vi "test-DiffDrvPoseEst2-Test2.vi"(8 "error in (no error)":errorcluster) -> (0 "error out":errorcluster, 3 "Test Passed":bool)   [LabVIEW 2019]
uses:
  <vilib>/Rock Robotics/WPI/ThirdParty/JAS_Junk/TrajLib/Rotation2d_CreateAngle.vi
  <vilib>/Rock Robotics/WPI/ThirdParty/JAS_Junk/TrajLib/MatBuilder_Create.vi
  <vilib>/Rock Robotics/SystemInterfaces/NetworkCommunication/NetComm_UsageReport_report.vi
  <vilib>/Rock Robotics/WPI/ThirdParty/JAS_Junk/TrajLib/Pose2d_TransformBy.vi
  <vilib>/Rock Robotics/WPI/ThirdParty/JAS_Junk/TrajLib/Translation2d_RotateBy.vi
  <vilib>/Rock Robotics/WPI/ThirdParty/JAS_Junk/TrajLib/Translation2d_Plus.vi
  <vilib>/Rock Robotics/WPI/ThirdParty/JAS_Junk/TrajLib/Rotation2d_Plus.vi
  <vilib>/Rock Robotics/WPI/ThirdParty/JAS_Junk/TrajLib/Pose2d_New_TRRO.vi
  <vilib>/Rock Robotics/WPI/ThirdParty/JAS_Junk/TrajLib/Rotation2d_RotateBy.vi
  <vilib>/Rock Robotics/WPI/ThirdParty/JAS_Junk/TrajLib/Rotation2d_CreateXY.vi
  <vilib>/Rock Robotics/WPI/ThirdParty/JAS_Junk/TrajLib/Util_CalcDist.vi
  <vilib>/Rock Robotics/WPI/ThirdParty/JAS_Junk/TrajLib/Globals/Util_LibraryGlobals.vi
  <vilib>/Rock Robotics/WPI/ThirdParty/JAS_Junk/TrajLib/Trajectory_Library.lvlib
panel:
  out "max x error":dbl
  out "max y err":dbl
  out "Y Error":dbl[](array[numeric])
  out "X error":dbl[](array[numeric])
  out "Total":i32
  out "Total passed":i32
  out "Sub error":bool
  out "End Y pos passed":bool
  out "End X pos passed":bool
  out "AddVisionCount":i32
  out "TotalTImeSecs 2":dbl
  out "BenchProcessing \nTimer Per Pass":dbl
  out "BenchTotalTime":dbl
  out "BenchTotalPasses":dbl
  out "MaxErrPassed":bool
  out "MeanPassed":bool
  out "ErrorSumNormalized":dbl
  out "Error Sum":dbl
  out "Max Error":dbl
  out "VIsionMeasCount":i32
  out "TotalTImeSecs":dbl
  out "Position Graph":cluster{dbl[], dbl[]}[](graph)
  out "PoseEst2NewErr":errorcluster
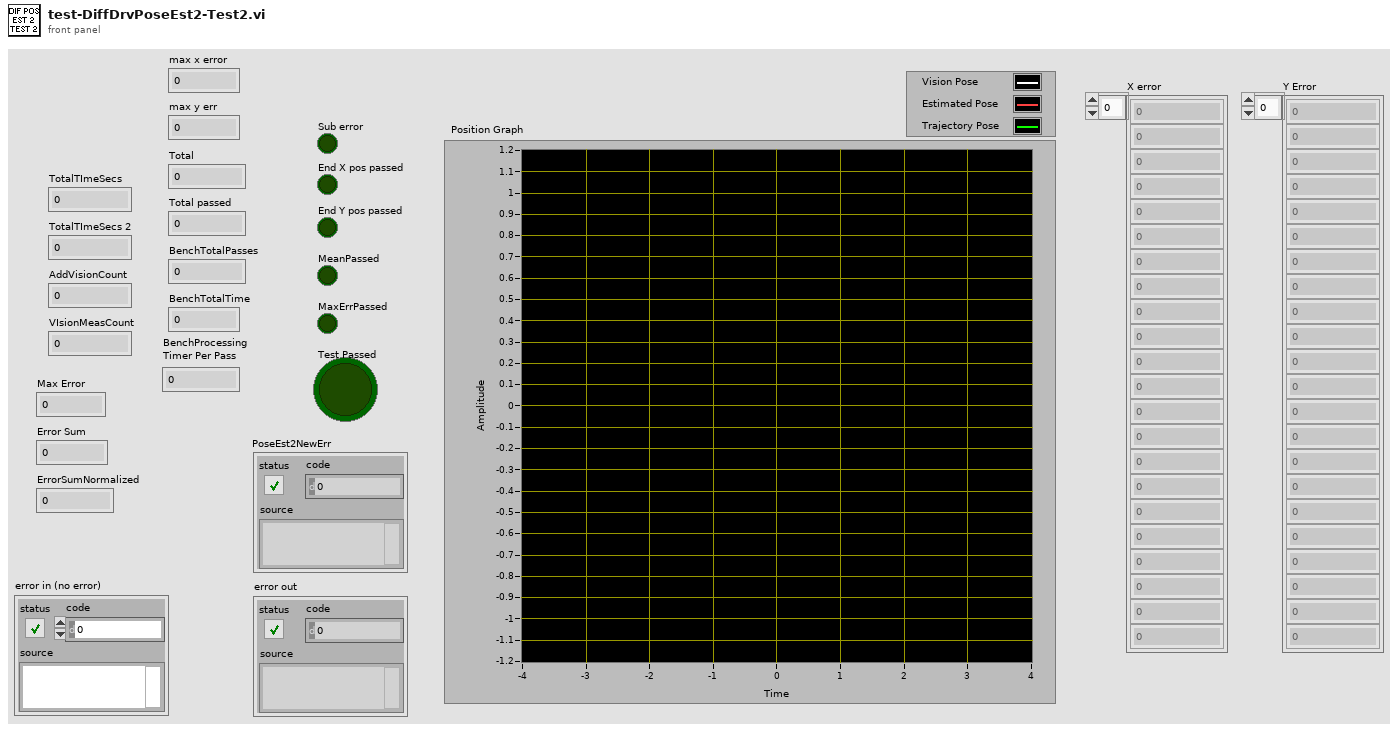
[diagram p1: front panel]
types:
  T1 = typedef "Trajectory_Library.lvlib/POSE2D.ctl" = cluster{"TRANSLATION":T2, "ROTATION":T3}
  T2 = typedef "Trajectory_Library.lvlib/TRANSLATION2D.ctl" = cluster{"X":dbl, "Y":dbl}
  T3 = typedef "Trajectory_Library.lvlib/ROTATION2D.ctl" = cluster{"VALUE":dbl, "COS":dbl, "SIN":dbl}
  T4 = typedef "NI_Matrix.lvlib/RealMatrix.ctl" = dbl[][]
  T5 = typedef "Trajectory_Library.lvlib/TRAJ_CONFIG.ctl" = cluster{"MaxVelocity":dbl, "Max Acceleration":dbl, "StartVelocity":dbl, "End Velocity":dbl, "Reversed":bool, "Constraints":variant[]}
  T6 = typedef "Trajectory_Library.lvlib/DIFF_DRIVE_KINEMATICS.ctl" = cluster{"TrackWidth_Meters":dbl}
  T7 = typedef "Trajectory_Library.lvlib/DIFF_DRIVE_POSE_EST2.ctl" = cluster{"M_Vision_K":T4, "m_nominal_dT":dbl, "m_PrevTime_Sec":dbl, "Pose_Buffer":T8, "Diff_Drive_Kinematics":T6, "Diff_Drive_Odom_2":T9, "M_Q":T4}
  T8 = typedef "Trajectory_Library.lvlib/TIME_INTERPOLATABLE_VARIANT.ctl" = cluster{"TimeStamps":dbl[], "DataArray":variant[], "Min_TimeStamp":dbl, "Max_TimeStamp":dbl, "ItemCount":i32, "MaxBufferTime":dbl}
  T9 = typedef "Trajectory_Library.lvlib/DIFF_DRIVE_ODOM2.ctl" = cluster{"M_POSE_Meters":T1, "M_GyroOffset":T3, "M_PrevAngle":T3, "M_PrevLeftDist_M":dbl, "M_PrevRightDist_M":dbl, "M_InitLeftDist_M":dbl, "M_InitRightDist_M":dbl}
  T10 = typedef "Trajectory_Library.lvlib/TRAJECTORY.ctl" = cluster{"TotalTImeSecs":dbl, "States":T11[]}
  T11 = typedef "Trajectory_Library.lvlib/TRAJ_STATE.ctl" = cluster{"TimeSeconds":dbl, "Velocity":dbl, "Acceleration":dbl, "POSE":T1, "Curvature":dbl}
  T12 = typedef "Trajectory_Library.lvlib/TRANSFORM2D.ctl" = cluster{"TRANSLATION":T2, "ROTATION":T3, "xF":bool}
  T13 = cluster{"MaxErrPassed":bool, "MeanPassed":bool, "Error Sum":dbl, "ErrorSumNormalized":dbl, "Max Error":dbl, "AddVisionCount":i32, "VIsionApplyCount":i32, "BenchTotalPasses":dbl, "BenchTotalTime":dbl, "BenchProcessing \nTimer Per Pass":dbl, "TotalTImeSecs":dbl, "End X pos passed":bool, "End Y pos passed":bool, "Sub error":bool, "End X Dev":dbl, "End Y Dev":dbl}
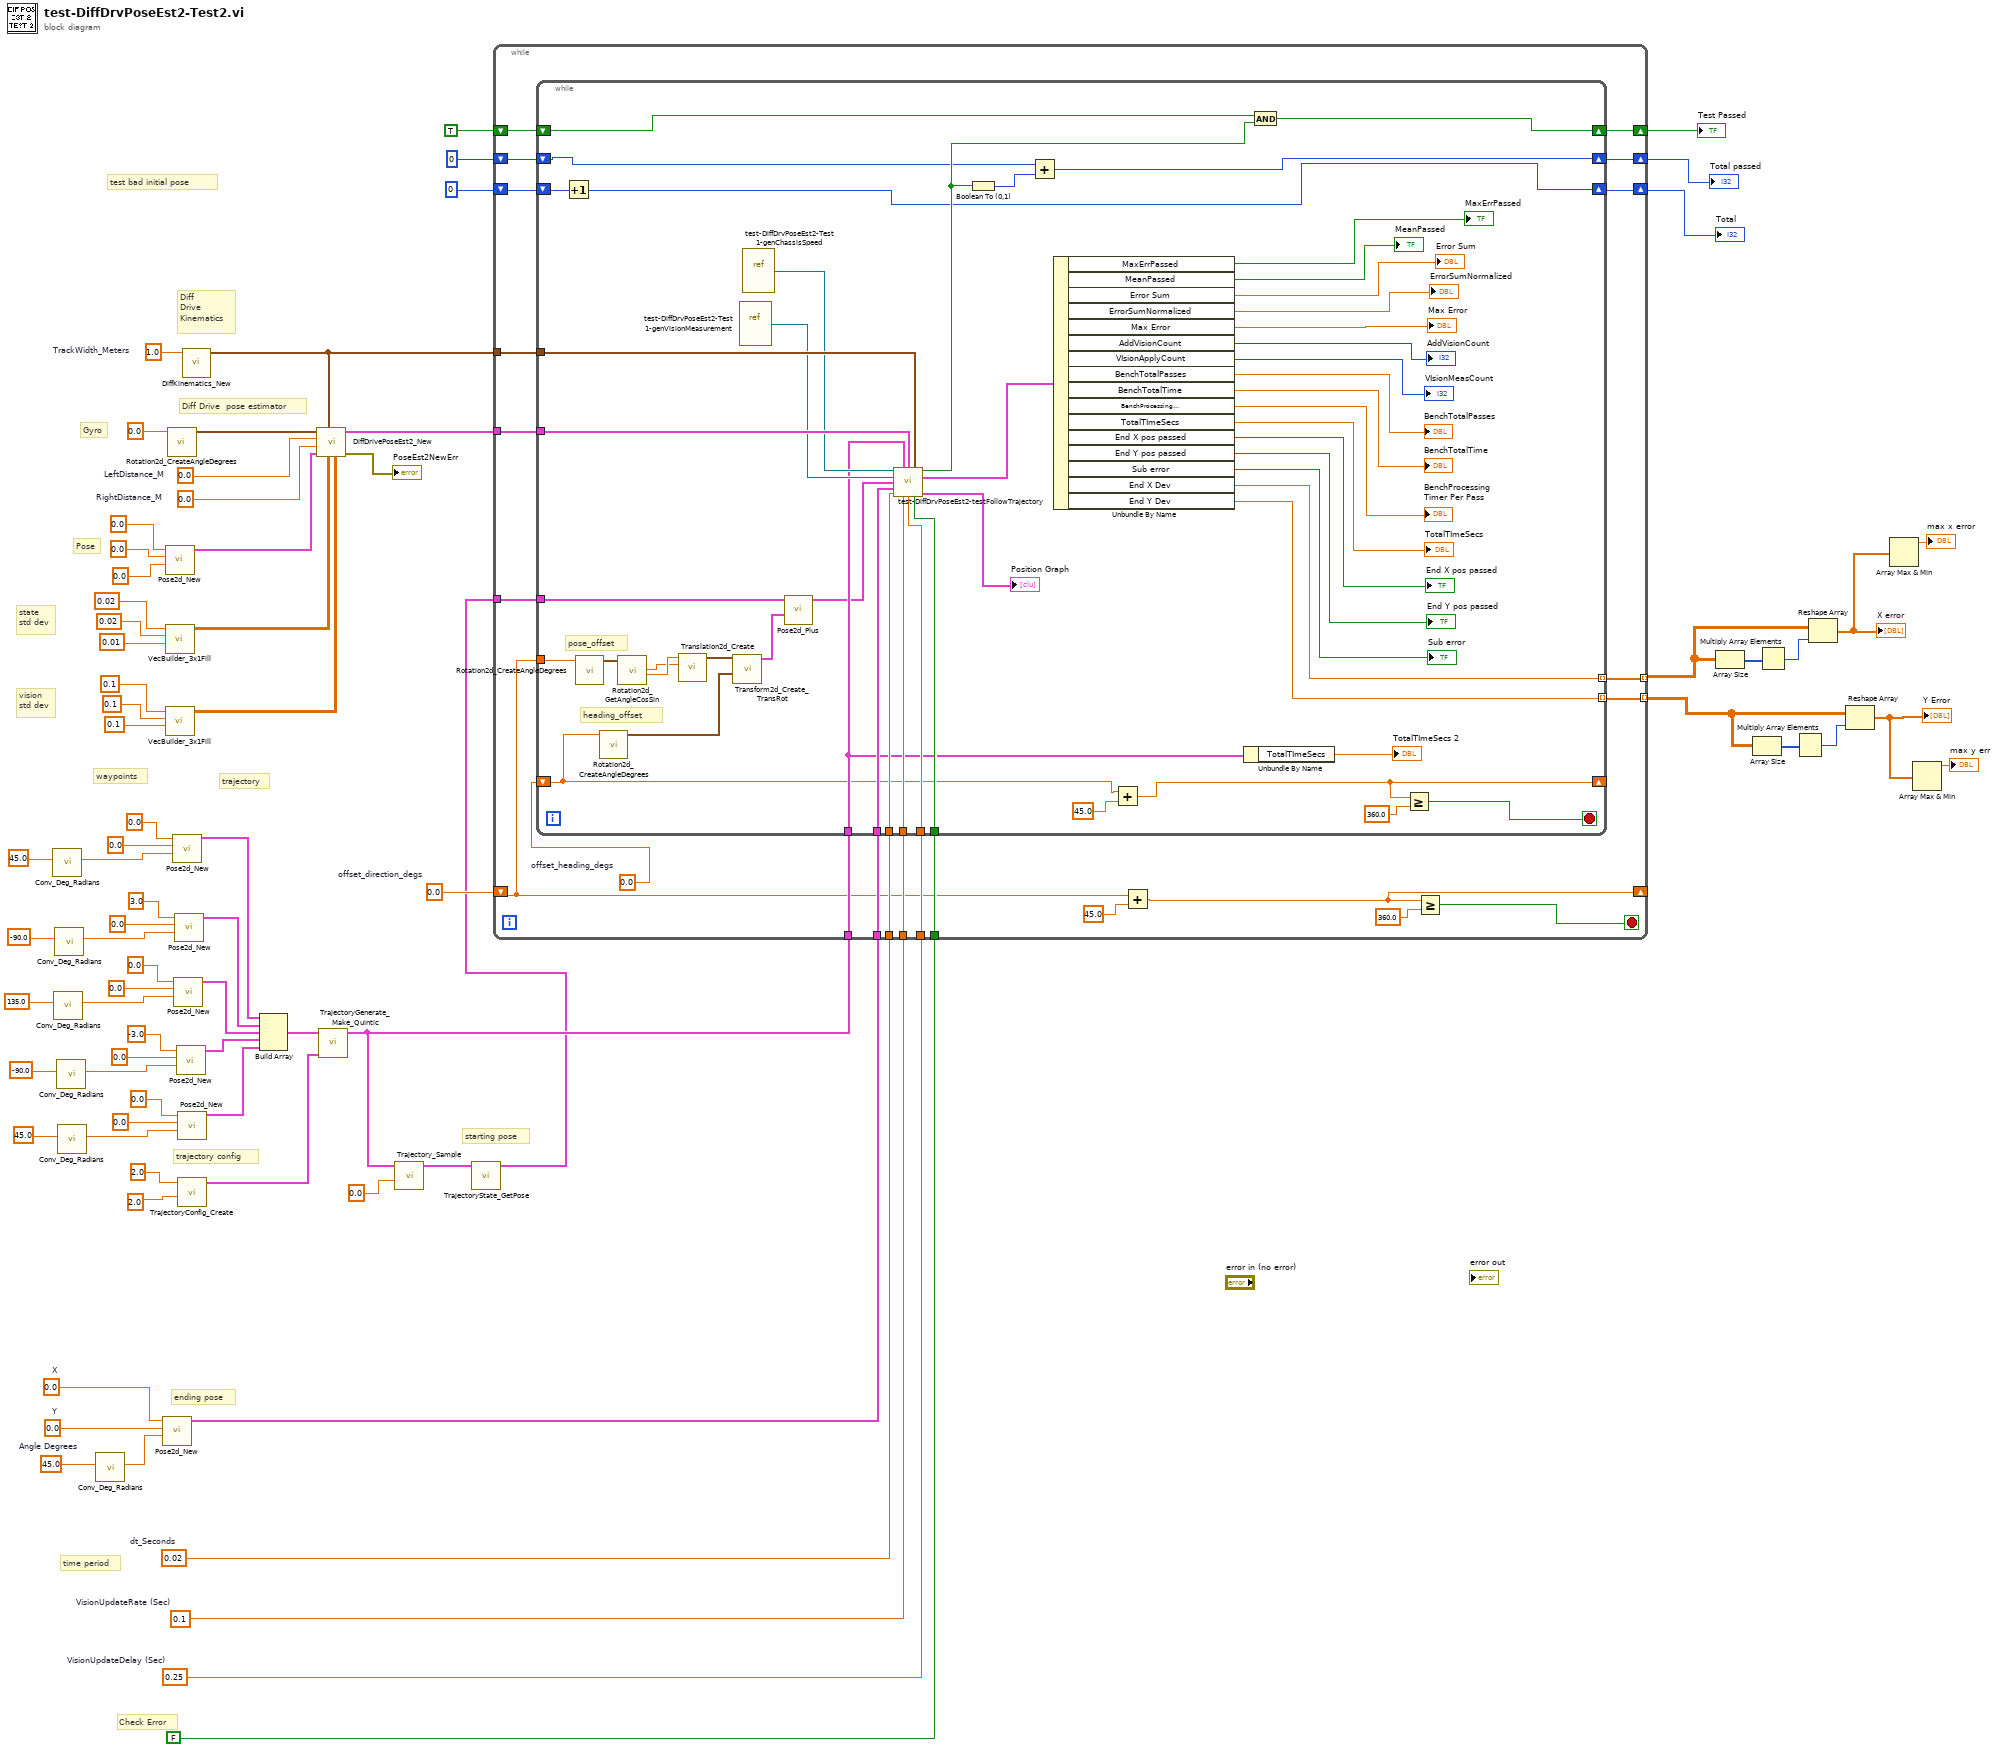
[diagram p0: block diagram]
diagram:
  w18 = 0.0  # offset_direction_degs
  w24 = 0.25  # VisionUpdateDelay (Sec)
  w25 = 0.1  # VisionUpdateRate (Sec)
  w30 = 0.0  # X
  w29 = 0.0  # Y
  w27 = 45.0  # Angle Degrees
  w38 = 1.0  # TrackWidth_Meters
  w41 = 0.0  # RightDistance_M
  w42 = 0.0  # LeftDistance_M
  w31 = 0.02  # dt_Seconds
  # "test bad initial pose"
  # "starting pose"
  # "Check Error"
  # "ending pose"
  # "state \nstd dev"
  # "Diff\nDrive\nKinematics"
  # "time period"
  # "vision \nstd dev"
  # "Pose"
  # "Gyro"
  # "Diff Drive  pose estimator"
  # "trajectory config"
  # "trajectory"
  # "waypoints"
  n1 = call <vilib>:"Conv_Deg_Radians.vi"("Degress"=45.0 ("Heading")) -> ("Radians"=w56:dbl)  [unwired: 10 in]
  n2 = call <vilib>:"Conv_Deg_Radians.vi"("Degress"=135.0 ("Heading")) -> ("Radians"=w64:dbl)  [unwired: 10 in]
  n3 = call <vilib>:"Conv_Deg_Radians.vi"("Degress"=-90.0 ("Heading")) -> ("Radians"=w60:dbl)  [unwired: 10 in]
  n4 = call <vilib>:"Conv_Deg_Radians.vi"("Degress"=-90.0 ("Heading")) -> ("Radians"=w68:dbl)  [unwired: 10 in]
  n5 = call <vilib>:"Conv_Deg_Radians.vi"("Degress"=45.0 ("Heading")) -> ("Radians"=w72:dbl)  [unwired: 10 in]
  n6 = call <vilib>:"Conv_Deg_Radians.vi"("Degress"=w27) -> ("Radians"=w28:dbl)  [unwired: 10 in]
  n7 = call <vilib>:"Pose2d_New.vi"("Heading"=w28, "Y"=w29, "X"=w30) -> ("out POSe"=w26:T1)  [unwired: 8 in]
  n8 = call <vilib>:"Pose2d_New.vi"("Heading"=0.0, "Y"=0.0, "X"=0.0) -> ("out POSe"=w40:T1)  [unwired: 8 in]
  n9 = call <vilib>:"VecBuilder_3x1Fill.vi"("R2"=0.01 ("element"), "R1"=0.02 ("element"), "R0"=0.02 ("element")) -> ("output matrix"=w34:T4)  [unwired: 8 in]
  n10 = call <vilib>:"VecBuilder_3x1Fill.vi"("R2"=0.1 ("element"), "R1"=0.1 ("element"), "R0"=0.1 ("element")) -> ("output matrix"=w33:T4)  [unwired: 8 in]
  n11 = call <vilib>:"Rotation2d_CreateAngleDegrees.vi"("Angle_Degrees"=0.0) -> ("ROTATION"=w39:T3)  [unwired: 10 in]
  n12 = call <vilib>:"Pose2d_New.vi"("Heading"=w56, "Y"=0.0, "X"=0.0) -> ("out POSe"=w55:T1)  [unwired: 8 in]
  n13 = call <vilib>:"Pose2d_New.vi"("Heading"=w64, "Y"=0.0, "X"=0.0) -> ("out POSe"=w52:T1)  [unwired: 8 in]
  n14 = call <vilib>:"Pose2d_New.vi"("Heading"=w60, "Y"=0.0, "X"=3.0) -> ("out POSe"=w53:T1)  [unwired: 8 in]
  n15 = call <vilib>:"Pose2d_New.vi"("Heading"=w68, "Y"=0.0, "X"=-3.0) -> ("out POSe"=w51:T1)  [unwired: 8 in]
  n16 = call <vilib>:"Pose2d_New.vi"("Heading"=w72, "Y"=0.0, "X"=0.0) -> ("out POSe"=w77:T1)  [unwired: 8 in]
  n17 = call <vilib>:"TrajectoryConfig_Create.vi"("MaxAcceleration"=2.0, "MaxVelocity"=2.0) -> ("TRAJECTORY_CONFIG"=w74:T5)  [unwired: 9 in]
  n18 = call <vilib>:"DiffKinematics_New.vi"("TrackWidth_Meters"=w38) -> ("DIFF_DRIVE_KINEMATICS"=w22:T6)  [unwired: 10 in]
  n19 = Build Array(w55, w53, w52, w51, w77) -> (w75:T1[])
  n20 = call <vilib>:"DiffDrivePoseEst2_New.vi"("VisionMeasurementStdDevs"=w33, "StateStdDevs"=w34, "DIFF_DRIVE_KINEMATICS"=w22, "InitialPose"=w40, "RightDistance_M"=w41, "LeftDistance_M"=w42, "gyroAngle"=w39) -> ("Error"=→"PoseEst2NewErr":errorcluster, "DiffDrivePoseEstimate"=w32:T7)  [unwired: 3 in]
  n21 = call <vilib>:"TrajectoryGenerate_Make_Quintic.vi"("traj_config"=w74, "waypointPOSE"=w75) -> ("TRAJECTORY"=w21:T10)  [unwired: 8 in, 1 out]
  n22 = call <vilib>:"Trajectory_Sample.vi"("Time"=0.0, "InputTRAJECTORY"=w21) -> ("OutputTRAJ_STATE"=w19:T11)  [unwired: 9 in]
  n23 = call <vilib>:"TrajectoryState_GetPose.vi"("TRAJ_STATE"=w19) -> ("TrajStatePose"=w17:T1)  [unwired: 10 in]
  n24 = while {
    tunnel: w32 -> [w102]
    tunnel: w31 -> [w101]
    tunnel: w26 -> [w100]
    tunnel: w25 -> [w99]
    tunnel: w24 -> [w98]
    tunnel: FALSE -> [w97]
    tunnel: w22 -> [w96]
    tunnel: w21 -> [w95]
    shift-right: [w90] -> _
    shift-left: w18 -> [w88]
    tunnel: w17 -> [w89]
    shift-right: [w86] -> w15
    shift-left: TRUE -> [w87]
    shift-right: [w84] -> w13
    shift-left: 0 -> [w85]
    shift-right: [w82] -> w11
    shift-left: 0 -> [w83]
    tunnel: [w81] -> w9 mode=indexing
    tunnel: [w80] -> w5 mode=indexing
    stop <- w92 stop-if-true
    w91 = 0.0  # offset_heading_degs
    n25 = while {
      tunnel: w102 -> [w153]
      tunnel: w101 -> [w152]
      tunnel: w100 -> [w151]
      tunnel: w99 -> [w150]
      tunnel: w98 -> [w149]
      tunnel: w97 -> [w147]
      tunnel: w96 -> [w146]
      tunnel: w95 -> [w128]
      shift-right: [w123] -> _
      shift-left: w91 -> [w121]
      tunnel: w89 -> [w114]
      tunnel: w88 -> [w119]
      shift-right: [w111] -> w86
      shift-left: w87 -> [w112]
      shift-right: [w107] -> w84
      shift-left: w85 -> [w109]
      shift-right: [w105] -> w82
      shift-left: w83 -> [w106]
      tunnel: [w104] -> w81 mode=indexing
      tunnel: [w103] -> w80 mode=indexing
      stop <- w124 stop-if-true
      # "heading_offset"
      # "pose_offset"
      n26 = Increment(x=w106) -> (x+1=w105:i32)
      n27 = call <vilib>:"Rotation2d_CreateAngleDegrees.vi"("Angle_Degrees"=w119) -> ("ROTATION"=w120:T3)  [unwired: 10 in]
      n28 = call <vilib>:"Rotation2d_CreateAngleDegrees.vi"("Angle_Degrees"=w121) -> ("ROTATION"=w116:T3)  [unwired: 10 in]
      n29 = call <vilib>:"Rotation2d_GetAngleCosSin.vi"("in ROTATION"=w120) -> ("Cosine"=w118:dbl, "Sine"=w117:dbl)  [unwired: 8 in, 1 out]
      n30 = call <vilib>:"Translation2d_Create.vi"("Y"=w117, "X"=w118) -> ("TRANSLATION"=w122:T2)  [unwired: 9 in]
      n31 = call <vilib>:"Transform2d_Create_TransRot.vi"("ROTATION"=w116, "TRANSLATION"=w122) -> ("TRANSFORM"=w115:T12)  [unwired: 9 in]
      n32 = vi-ref "test-DiffDrvPoseEst2-Test1-genVisionMeasurement.vi"() -> (w144:refnum<vi>)
      n33 = vi-ref "test-DiffDrvPoseEst2-Test1-genChassisSpeed.vi"() -> (w145:refnum<vi>)
      n34 = call <vilib>:"Pose2d_Plus.vi"("other TRANSFORM"=w115, "in POSE"=w114) -> ("out POSE"=w113:T1)  [unwired: 9 in]
      n35 = call "test-DiffDrvPoseEst2-testFollowTrajectory.vi"("chassisSpeedsGenerator"=w145, "TRAJECTORY"=w128, "DiffDrivePoseEstimate"=w153, "DIFF_DRIVE_KINEMATICS"=w146, "genVisionMeasurement"=w144, "StartingPose"=w113, "EndingPose"=w151, "dt_Seconds"=w152, "VisionUpdateRate"=w150, "VisionUpdateDelay"=w149, "CheckError"=w147) -> ("Test Passed"=w110:bool, "Output Data"=w142:T13, "DataForGraph"=→"Position Graph":cluster{dbl[], dbl[]}[])  [unwired: 2 in]
      n36 = Boolean To (0,1)(Boolean=w110) -> (0, 1=w108:i16)
      n37 = Add(x=w109, y=w108) -> (x+y=w107:i32)
      n38 = Unbundle By Name(w142) -> ("MaxErrPassed"=→"MaxErrPassed":bool, "MeanPassed"=→"MeanPassed":bool, "Error Sum"=→"Error Sum":dbl, "ErrorSumNormalized"=→"ErrorSumNormalized":dbl, "Max Error"=→"Max Error":dbl, "AddVisionCount"=→"AddVisionCount":i32, "VIsionApplyCount"=→"VIsionMeasCount":i32, "BenchTotalPasses"=→"BenchTotalPasses":dbl, "BenchTotalTime"=→"BenchTotalTime":dbl, "BenchProcessing \nTimer Per Pass"=→"BenchProcessing \nTimer Per Pass":dbl, "TotalTImeSecs"=→"TotalTImeSecs":dbl, "End X pos passed"=→"End X pos passed":bool, "End Y pos passed"=→"End Y pos passed":bool, "Sub error"=→"Sub error":bool, "End X Dev"=w104:dbl, "End Y Dev"=w103:dbl)
      n39 = Add(x=w121, y=45.0) -> (x+y=w123:dbl)
      n40 = Unbundle By Name(w128) -> ("TotalTImeSecs"=→"TotalTImeSecs 2":dbl)
      n41 = And(x=w112, y=w110) -> (x .and. y?=w111:bool)
      n42 = Greater Or Equal?(x=w123, y=360.0) -> (x >= y?=w124:bool)
    }
    n43 = Add(x=w88, y=45.0) -> (x+y=w90:dbl)
    n44 = Greater Or Equal?(x=w90, y=360.0) -> (x >= y?=w92:bool)
  }
  "Test Passed" <- w15
  "Total passed" <- w13
  "Total" <- w11
  n45 = Array Size(array=w9) -> (size(s)=w10:i32[])
  n46 = Array Size(array=w5) -> (size(s)=w7:i32[])
  n47 = Multiply Array Elements(1:w10) -> (0:w8:i32)
  n48 = Multiply Array Elements(1:w7) -> (0:w6:i32)
  n49 = Reshape Array(w9, w8) -> (w4:dbl[])
  "X error" <- w4
  n50 = Reshape Array(w5, w6) -> (w3:dbl[])
  "Y Error" <- w3
  n51 = Array Max & Min(array=w4) -> (max value=→"max x error":dbl)  [unwired: 3 out]
  n52 = Array Max & Min(array=w3) -> (max value=→"max y err":dbl)  [unwired: 3 out]
